vi "discharge.vi"() -> ()   [LabVIEW 2022 SP3]
panel:
  in  "Sample Rate [Hz]":dbl=5000.0
  in  "Delay between files [s]":dbl=3.0 caption="Delay Time (s)"
  in  "Number of Samples":i32=20000
  in  "Num files":i32=1000
  in  "File base name":string="turbombar_powfb_xyzcool"
  in  "Directory path":path=path "D:/data/20190626/bead1/spinning/pramp/SF6/rga/discharge_main"
  in  "Electrode settings:":T1={"Electrode to sweep:"=3, "amplitude (V)"=2.0, "frequency (Hz)"=41.0, "offset (V)"=0.0, "Sweep electrode?"=TRUE, "Control DDS"=TRUE}
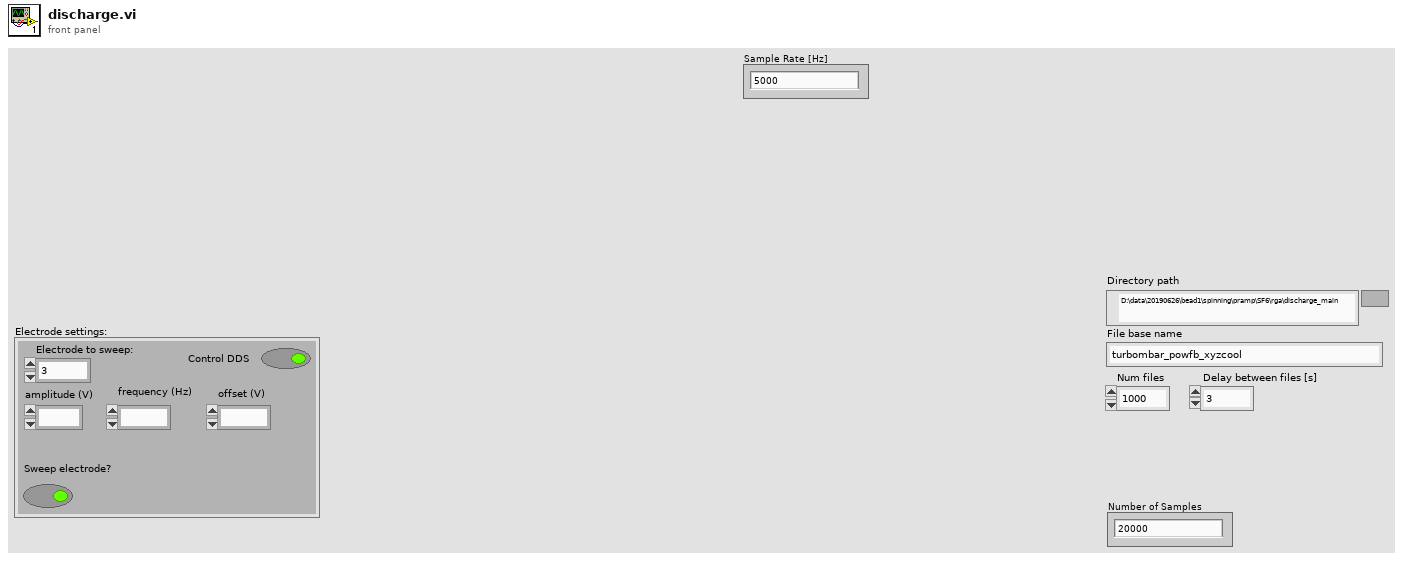
[diagram p1: front panel]
types:
  T1 = cluster{"Electrode to sweep:":i32, "amplitude (V)":ext, "frequency (Hz)":ext, "offset (V)":ext, "Sweep electrode?":bool, "Control DDS":bool}
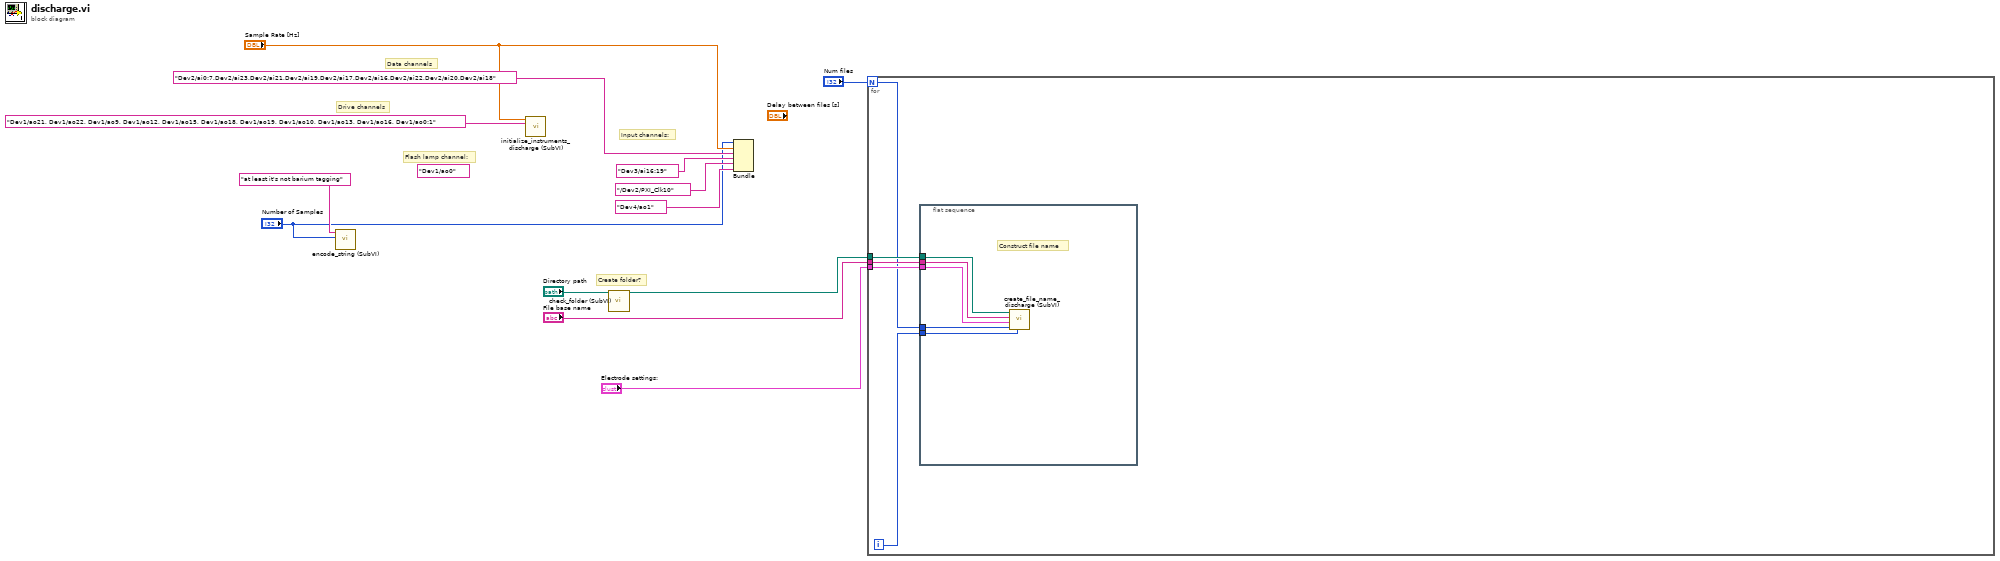
[diagram p0: block diagram]
diagram:
  (unwired) tag "Dev1/ao0" ("Output channel (for flashing)")
  # "Drive channels"
  # "Data channels"
  # "Input channels:"
  # "Flash lamp channel:"
  # "Create folder?"
  n1 = call "encode_string (SubVI).vi"("nsamp"="Number of Samples", "encode_string"="at least it's not barium tagging") -> ()  [unwired: 8 in, 2 out]
  n2 = call "initialize_instruments_discharge (SubVI).vi"("Sample rate"="Sample Rate [Hz]", "Electrode outupt channels"=tag "Dev1/ao21, Dev1/ao22, Dev1/ao9, Dev1/ao12, Dev1/ao15, Dev1/ao18, Dev1/ao19, Dev1/ao10, Dev1/ao13, Dev1/ao16, Dev1/ao0:1" ("Output channel (for flashing)")) -> ()  [unwired: 12 in, 2 out]
  n3 = call "check_folder (SubVI).vi"("path in"="Directory path") -> ("path out"=w3:path)  [unwired: 10 in]
  n4 = Bundle("Number of Samples"="Number of Samples", "Sample Rate [Hz]"="Sample Rate [Hz]", "Physical Channels (Position signals)"=tag "Dev2/ai0:7,Dev2/ai23,Dev2/ai21,Dev2/ai19,Dev2/ai17,Dev2/ai16,Dev2/ai22,Dev2/ai20,Dev2/ai18", "Physical Channel (drive signals)"=tag "Dev3/ai16:19", "Sample Clock Source"=tag "/Dev2/PXI_Clk10", "Physical Channel (drive signals)"=tag "Dev4/ao1") -> ()  [unwired: 1 in, 1 out]
  n5 = for {
    N: "Num files" -> [w15]
    tunnel: w3 -> [w18]
    tunnel: "File base name" -> [w17]
    tunnel: "Electrode settings:" -> [w16]
    i -> [w14]
    n6 = flat-sequence {
      tunnel: w18 -> [w23]
      tunnel: w17 -> [w22]
      tunnel: w16 -> [w21]
      tunnel: w15 -> [w20]
      tunnel: w14 -> [w19]
      frame #0 {
        # "Construct file name"
        n7 = call "create_file_name_discharge (SubVI).vi"("file_idx"=w19, "num files"=w20, "Electrode settings:"=w21, "base name"=w22, "base_path"=w23) -> ()  [unwired: 6 in, 1 out]
      }
    }
  }
